vi "Inst.Krohn-Hite-7008.ReplaceChannelProperty.vi"(10 "channelProperties":T2 {"channel" min=1 max=8 step=1}, 11 "allChannelProperties":T1 {"channel" min=1 max=8 step=1}) -> (3 "allChannelProperties":T1 {"channel" min=1 max=8 step=1})   [LabVIEW 2019, in "Inst.KH7008.lvlib" / "Inst.Krohn-Hite-7008.lvclass"]
uses:
  Inst.Krohn-Hite-7008.lvclass
  KH7008/typedefs/allChannelProperties--Array.ctl
  KH7008/typedefs/channelProperties--Cluster.ctl
  KH7008/typedefs/channel--numeric.ctl
  KH7008/typedefs/gain--enum.ctl
  KH7008/typedefs/Input--Enum.ctl
  KH7008/typedefs/shunt--enum.ctl
  KH7008/typedefs/couple--Enum.ctl
  KH7008/typedefs/Filter--Enum.ctl
  KH7008/KH7008.lvlib
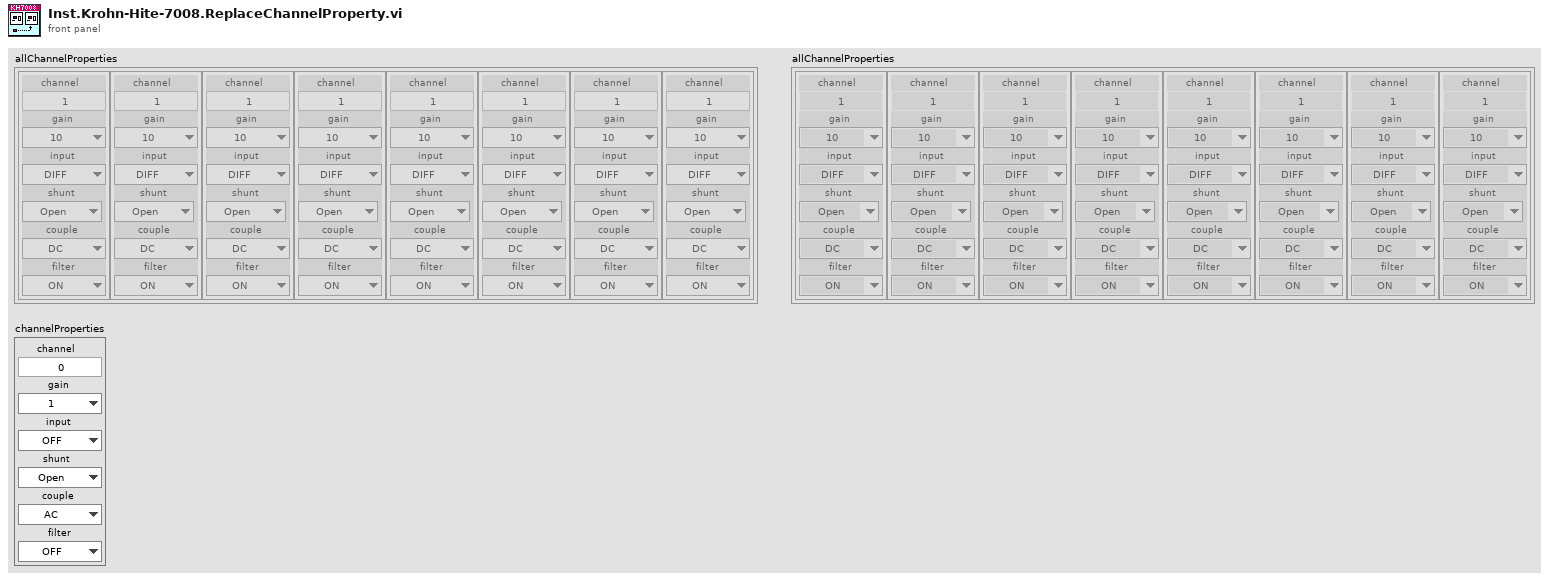
[diagram p1: front panel]
types:
  T1 = typedef "KH7008.lvlib/allChannelProperties--Array.ctl" = T2[]
  T2 = typedef "KH7008.lvlib/channelProperties--Cluster.ctl" = cluster{"channel":T3, "gain":T4, "input":T5, "shunt":T6, "couple":T7, "filter":T8}
  T3 = typedef "KH7008.lvlib/channel--numeric.ctl" = u16
  T4 = typedef "KH7008.lvlib/gain--enum.ctl" = enum16{"1", "10", "100", "1000"}
  T5 = typedef "KH7008.lvlib/input--enum.ctl" = enum16{"OFF", "SE+", "SE-", "DIFF"}
  T6 = typedef "KH7008.lvlib/shunt--enum.ctl" = enum16{"Open", "50", "500", "5k", "50k", "10M"}
  T7 = typedef "KH7008.lvlib/couple--enum.ctl" = enum16{"AC", "DC"}
  T8 = typedef "KH7008.lvlib/filter--enum.ctl" = enum16{"OFF", "ON"}
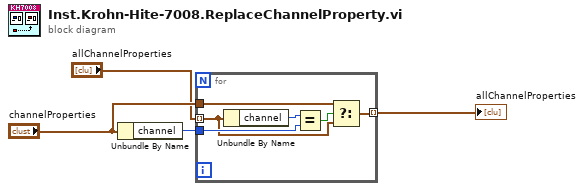
[diagram p0: block diagram]
diagram:
  n1 = Unbundle By Name("channelProperties") -> ("channel"=w2:T3)
  n2 = for {
    tunnel: "allChannelProperties" -> [w6] mode=indexing
    tunnel: w2 -> [w9]
    tunnel: "channelProperties" -> [w7]
    tunnel: [w5] -> w4 mode=indexing
    n3 = Unbundle By Name(w6) -> ("channel"=w10:T3)
    n4 = Equal?(x=w10, y=w9) -> (x = y?=w8:bool)
    n5 = Select(t=w7, s=w8, f=w6) -> (s? t:f=w5:T2)
  }
  "allChannelProperties" <- w4
